vi "DLC validate.vi"(8 "error in":errorcluster, 11 "in":i32) -> (0 "error out":errorcluster, 2 "invalid?":bool, 3 "out":i32)   [LabVIEW 2025, in "CAN-LIN Frame Generator UI.lvlib"]
uses:
  CAN-LIN Frame Generator UI.lvlib
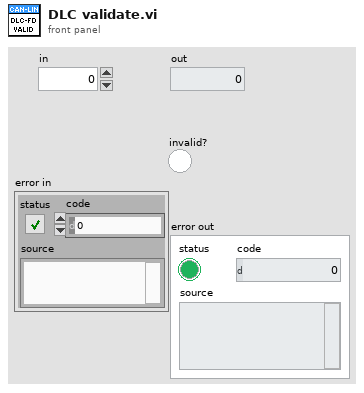
[diagram p1: front panel]
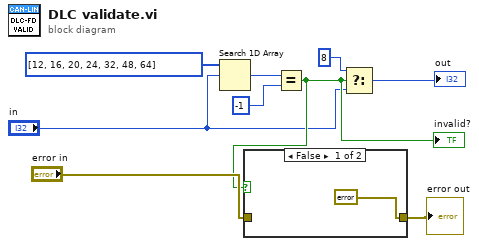
[diagram p0: block diagram]
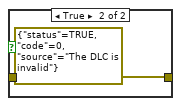
[diagram p2: hidden frame]
diagram:
  n1 = Search 1D Array(1D array=i32[] [12, 16, 20, 24, 32, 48, 64], element="in") -> (index of element=w3:i32)  [unwired: 1 in]
  n2 = Equal?(x=w3, y=-1) -> (x = y?=w7:bool)
  "invalid?" <- w7
  n3 = case shown="False" w7 {
    tunnel: "error in" -> [_ _]
    tunnel: [errorcluster {"status"=FALSE, "code"=0, "source"=""} ("error constant") errorcluster {"status"=TRUE, "code"=0, "source"="The DLC is invalid"} ("error constant")] -> w9
    frame False {
    }
    frame True {
    }
  }
  "error out" <- w9
  n4 = Select(t=8, s=w7, f="in") -> (s? t:f=→"out":i32)
